vi "Test_WriteValue_ActorReceives_ValuesMatch.vi"(8 "error in (no error)":errorcluster, 11 "TestCase in":refnum<class "TestActorMessageTransport.lvclass">) -> (0 "error out":errorcluster, 3 "TestCase out":refnum<class "TestActorMessageTransport.lvclass">)   [LabVIEW 2017, in "TestActorMessageTransport.lvclass"]
uses:
  TestActorMessageTransport.lvclass
  <vilib>/ActorFramework/Actor/Actor.lvclass
  MockNotificationMsg/MockNotificationMsg.lvclass/MockNotificationMsg.ctl
  Source/Concrete/ActorMessageTransport/ActorMessageTransport.lvclass/ActorMessageTransport.ctl
  <vilib>/ActorFramework/Message Enqueuer/Message Enqueuer.lvclass/Message Enqueuer.ctl
  <vilib>/ActorFramework/Message Enqueuer/Equals Not A Refnum.vi
  <vilib>/ActorFramework/Message Enqueuer/Enqueue.vi
  MockNotificationMsg/MockNotificationMsg.lvclass
  C:/Git/composed-transport/Source/Concrete/ActorMessageTransport/Notification Msg/Notification Msg.lvclass
  Source/Concrete/ActorMessageTransport/ActorMessageTransport.lvclass
  C:/Git/composed-transport/Source/ITransport/ITransport.lvclass
  <vilib>/ActorFramework/Stop Msg/Stop Msg.lvclass
  C:/Program Files (x86)/National Instruments/LabVIEW 2017/vi.lib/ActorFramework/Message/Message.lvclass
  <vilib>/Utility/error.llb/Error Cluster From Error Code.vi
  <vilib>/ActorFramework/Message Priority Queue/Priority Enqueue.vi
  <vilib>/ActorFramework/Message Enqueuer/Message Enqueuer.lvclass
  Source/Concrete/ActorMessageTransport/Notification Msg/Notification Msg.lvclass
  Source/ITransport/ITransport.lvclass
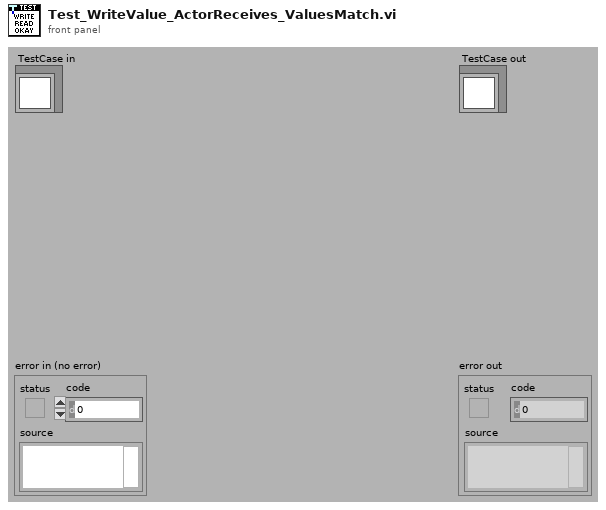
[diagram p1: front panel]
types:
  T1 = cluster{"Datum Name":string, "Value":variant, "Publication Time":timestamp}
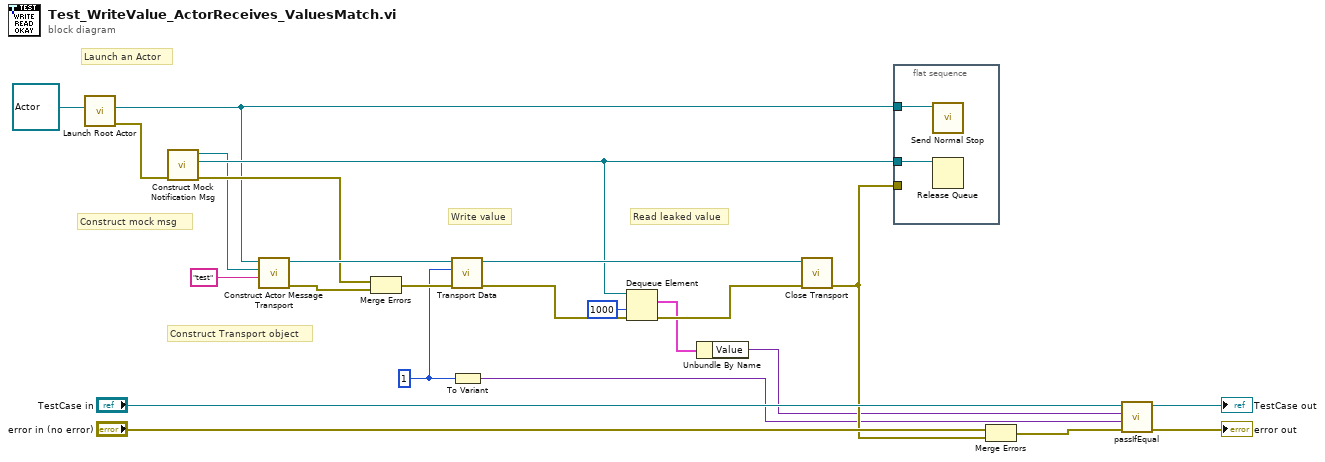
[diagram p0: block diagram]
diagram:
  w2 = 1
  # "Construct Transport object"
  # "Construct mock msg"
  # "Launch an Actor"
  # "Read leaked value"
  # "Write value"
  n1 = call <vilib>:"Launch Root Actor.vi"("Actor"=refnum<class "Actor.lvclass"> refnum) -> ("error out"=w5:errorcluster, "Actor's Enqueuer"=w7:refnum<class "Message Enqueuer.lvclass">)  [unwired: 9 in]
  n2 = call "Construct Mock Notification Msg.vi"("error in (no error)"=w5) -> ("error out"=w23:errorcluster, "Data leak test queue"=w10:refnum<queue>, "MockNotificationMsg out"=w8:refnum<class "MockNotificationMsg.lvclass">)  [unwired: 8 in]
  n3 = call "Construct Actor Message Transport.vi"("Datum Name"="test", "Notification Msg"=w8, "Message Enqueuer in"=w7) -> ("error out"=w17:errorcluster, "ActorMessageTransport"=w24:refnum<class "ActorMessageTransport.lvclass">)  [unwired: 7 in]
  n4 = Merge Errors(w23, w17) -> (w4:errorcluster)
  n5 = call "Transport Data.vi"("error in (no error)"=w4, "Value"=w2, "ITransport in"=w24) -> ("error out"=w13:errorcluster, "ITransport out"=w16:refnum<class "ActorMessageTransport.lvclass">)  [unwired: 7 in]
  n6 = To Variant(anything=w2) -> (Variant=w1:variant)
  n7 = Dequeue Element(queue=w10, timeout in ms (-1)=1000, error in (no error)=w13) -> (element=w6:T1, error out=w12:errorcluster)  [unwired: 2 out]
  n8 = Unbundle By Name(w6) -> ("Value"=w3:variant)
  n9 = call-dynamic "Close Transport.vi"("error in (no error)"=w12, "ITransport in"=w16) -> ("error out"=w9:errorcluster)  [unwired: 9 in]
  n10 = flat-sequence {
    tunnel: w10 -> [w26]
    tunnel: w7 -> [w25]
    tunnel: w9 -> [_]
    frame #0 {
      n11 = call <vilib>:"Send Normal Stop.vi"("Message Enqueuer"=w25) -> ()  [unwired: 10 in, 1 out]
      n12 = Release Queue(queue=w26) -> ()  [unwired: 2 in, 3 out]
    }
  }
  n13 = Merge Errors("error in (no error)", w9) -> (w18:errorcluster)
  n14 = call-dynamic "passIfEqual.vi"("error in (no error)"=w18, "y"=w1, "x"=w3, "TestCase in"="TestCase in") -> ("error out"=→"error out":errorcluster, "TestCase out"=→"TestCase out":refnum<class "TestActorMessageTransport.lvclass">)  [unwired: 6 in]
